vi "Write Meta Data.vi"(7 "Linked List ID":string, 8 "error in (no error)":errorcluster, 10 "Meta Data":string, 11 "Linked List Ref":refnum<data-value>) -> (0 "error out":errorcluster, 1 "Found?":bool, 3 "Linked List Ref out":refnum<data-value>)   [LabVIEW 2020, in "Linked Lists.lvlib" / "Linked List Ref.lvclass"]
uses:
  <vilib>/gpm_packages/@cs/linked-list/Source/Linked List/Linked List Ref/Linked List Ref.lvclass
  <vilib>/gpm_packages/@cs/linked-list/Source/Linked List/ILinkedList/ILinked List.lvclass
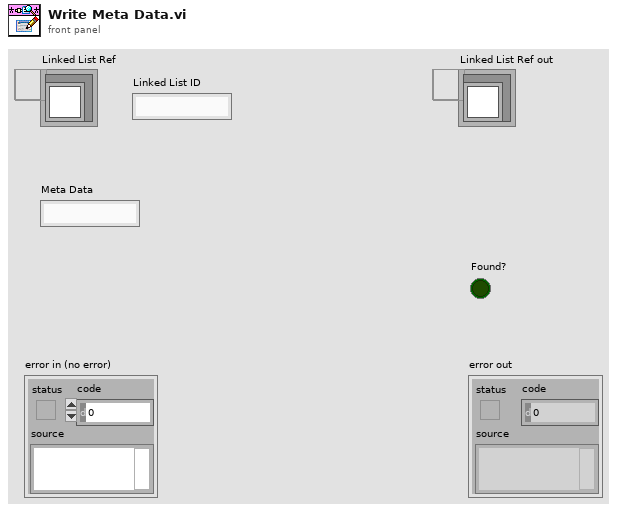
[diagram p1: front panel]
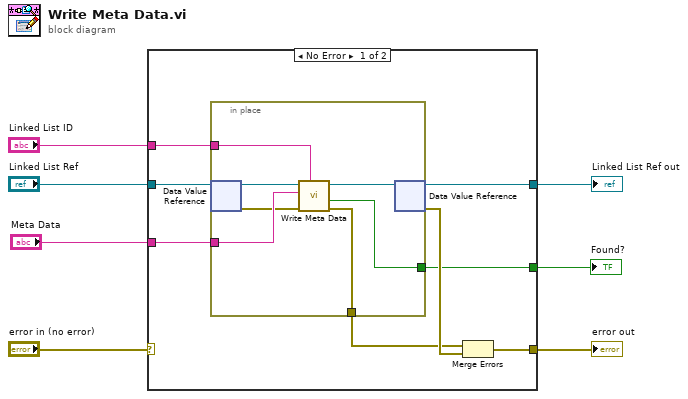
[diagram p0: block diagram]
diagram:
  n1 = case shown="No Error" "error in (no error)" {
    selector: "error in (no error)" -> [_ w24]
    tunnel: "Linked List Ref" -> [w15 w23]
    tunnel: "Linked List ID" -> [w14 _]
    tunnel: [w12 w24] -> w4
    tunnel: [w13 w23] -> w3
    tunnel: "Meta Data" -> [w9 _]
    tunnel: [w8 _] -> w1
    frame No Error {
      n2 = in-place {
        in-place-border: w14 -> [w22]
        in-place-border: [w17] -> w10
        in-place-border: w9 -> [w19]
        in-place-border: [w16] -> w8
        n3 = in-place-dvr #1(w15) -> (w21:refnum<class "ILinked List.lvclass">, w18:errorcluster)
        n4 = call-dynamic "Write Meta Data.vi"("Unique ID"=w22, "error in (no error)"=w18, "Meta Data"=w19, "ILinked List in"=w21) -> ("error out"=w17:errorcluster, "Found?"=w16:bool, "ILinked List out"=w20:refnum<class "ILinked List.lvclass">)  [unwired: 5 in]
        n5 = in-place-dvr #1(w20) -> (w13:refnum<data-value>, w11:errorcluster)
      }
      n6 = Merge Errors(w10, w11) -> (w12:errorcluster)
    }
    frame Error {
    }
  }
  "error out" <- w4
  "Linked List Ref out" <- w3
  "Found?" <- w1
